vi "WBRT Main.vi"() -> ()   [LabVIEW 2012]
doc: "Whirlybird Controller\n\nAuthor: Brandon Steele\n\nCopyright: Brigham Young University"
uses:
  Custom Controls/WBRT Filter Data.ctl
  Custom Controls/WBRT Filter Type.ctl
  Custom Controls/WBRT Setpoints.ctl
  Custom Controls/WBRT Gains.ctl
  <vilib>/Platform/TimedLoop/XDataNode/timing_clust.ctl
  <vilib>/Platform/TimedLoop/XDataNode/nitl_modes.ctl
  <vilib>/Platform/TimedLoop/XDataNode/wakeup.ctl
  <vilib>/Platform/TimedLoop/XDataNode/XDataNode.xnode
  <vilib>/Platform/TimedLoop/XDataNode/XDNodeRunTimeDep.lvlib
  <vilib>/vision/NI_Vision_Development_Module.lvlib
panel:
  in  "Zero Encoders":bool
  in  "Tab Control":T1(tab)
  out "Waveform\nChart":T2(graph)={"[0]"=-46.87203500802024, "[1]"=-28.440021241425494, "[2]"=-1.368001021739454, "[3]"=0.0, "[4]"=0.0, "[5]"=0.0, "[6]"=-0.58608, "[7]"=-4.542120000000001, "[8]"=-5.347980000000001, "[9]"=-0.5018779999999999, "[10]"=0.6305, "[11]"=-0.633022}
  out "dt (msec)":u32=67
  in  "Red or Hue Range":cluster{"Lower value":i32, "Upper value":i32}={"Lower value"=150, "Upper value"=255}
  in  "Green Range":cluster{"Lower value":i32, "Upper value":i32}={"Lower value"=0, "Upper value"=255}
  in  "Blue Range":cluster{"Lower value":i32, "Upper value":i32}={"Lower value"=0, "Upper value"=255}
  in  "Pixel Format":T3(ring)=enum."160 x 120 MJPG"
  in  "Compression":u32(slide)=85 scale=0.0..99.0
  in  "Frame Rate":u32(slide)=15 max=30 scale=0.0..30.0
  in  "Camera IP address":string="192.168.0.90"
  out "Centroid":cluster{"X Centroid":sgl, "Y Centroid":sgl}={"X Centroid"=78.86318, "Y Centroid"=61.304207} {"Y Centroid" format="%.2f"; "X Centroid" format="%.2f"}
  in  "Find Centroid":bool
  out "Image":T4(plugin-control)
  out "Error Chart":T5(graph)
  in  "Auto Zero?":bool
  in  "Delay (s)":dbl=30.0
  in  "Auto Shutdown":bool
  in  "Left Motor (0-100%)":dbl
  in  "Right Motor (0-100%)":dbl
  in  "Manual Motor Control":bool
  out "Left Motor Display":dbl=-1.2876027999998882
  out "Right Motor Display":dbl=-0.09379669999989915
  in  "Lock together":bool=TRUE
  in  "Save Data":bool
  out "Array Size":i32
  in  "Filter Data":T6={"Filter Enabled?"=FALSE, "Filter Type"=enum."Equi-Ripple", "Pass Frequency"=0.45000000000000007, "Stop Frequency (Equi-Ripple)"=0.125, "Order"=2, "Ripple (dB)"=2.0} {"Stop Frequency (Equi-Ripple)" format="%0.3f"; "Pass Frequency" format="%0.3f"}
  in  "Landing Factor\n(power reduction per loop)":dbl=0.1
  in  "Enable Camera":bool
  out "Camera \nerror codes":errorcluster
  in  "Spin up time (s)":dbl=2.0
  in  "Gains":T8
  in  "Commanded Values":T9
  in  "Start":bool
  in  "Stop":bool
  out "Running":bool
  out "Late?":bool
  out "Freq (Hz)":dbl=100.0
  out "dt (msec)":u32=10
  in  "Loop Rate (Hz)":dbl=100.0
  # "Color Segmentation Thresholds"
  # "Must be set before runtime"
  # "Run Mathscript Node"
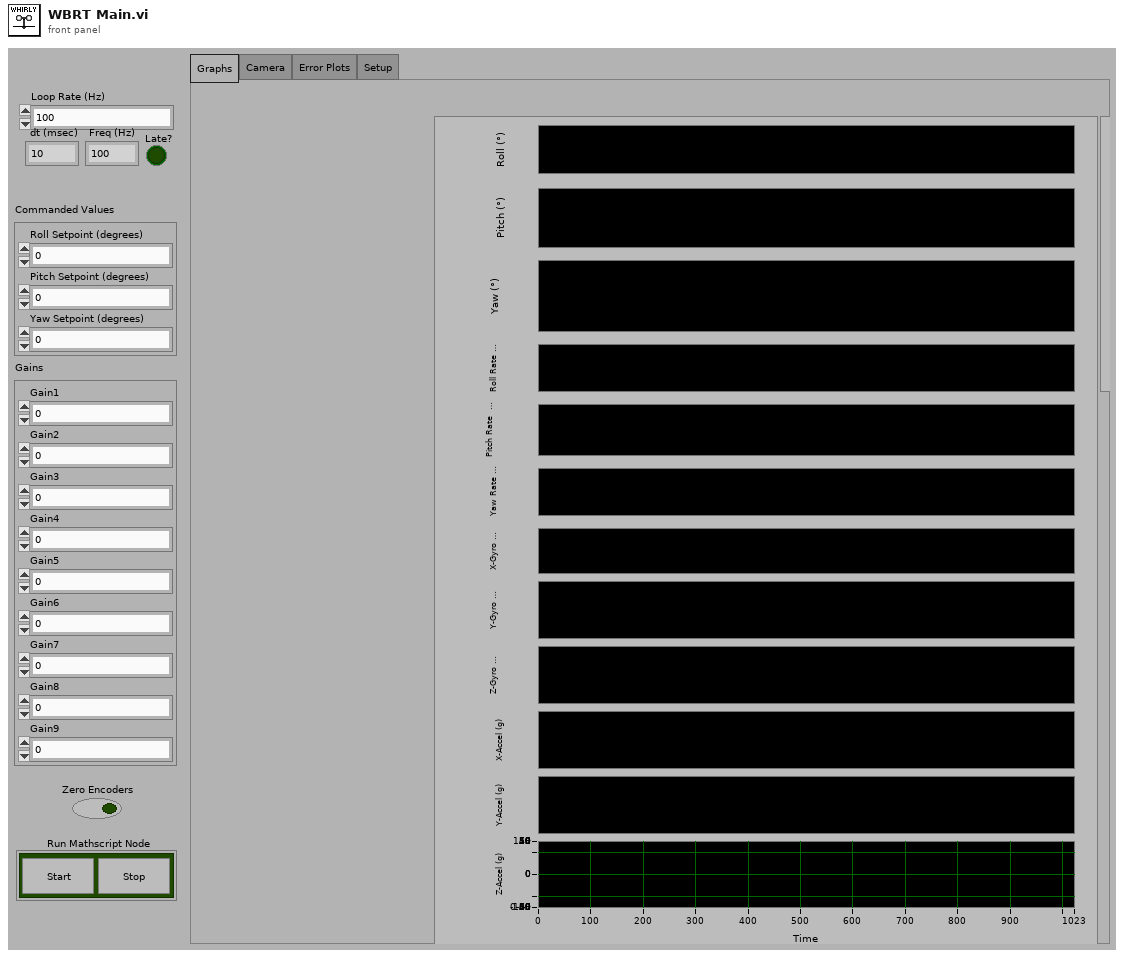
[diagram p1: front panel]
types:
  T1 = enum32{"Graphs", "Camera", "Error Plots", "Setup"}
  T2 = cluster{"[0]":dbl, "[1]":dbl, "[2]":dbl, "[3]":dbl, "[4]":dbl, "[5]":dbl, "[6]":dbl, "[7]":dbl, "[8]":dbl, "[9]":dbl, "[10]":dbl, "[11]":dbl}
  T3 = enum16{"640 x 480 MJPG", "320 x 240 MJPG", "160 x 120 MJPG"}
  T4 = typedef "IMAQ Image.ctl" = refnum<image>
  T5 = cluster{"[0]":dbl, "[1]":dbl, "[2]":dbl, "[3]":dbl}
  T6 = typedef "WBRT Filter Data.ctl" = cluster{"Filter Enabled?":bool, "Filter Type":T7, "Pass Frequency":dbl, "Stop Frequency (Equi-Ripple)":dbl, "Order":i32, "Ripple (dB)":dbl}
  T7 = typedef "WBRT Filter Type.ctl" = enum16{"Equi-Ripple", "Butterworth", "Chebyshev"}
  T8 = typedef "WBRT Gains.ctl" = cluster{"Gain1":dbl, "Gain2":dbl, "Gain3":dbl, "Gain4":dbl, "Gain5":dbl, "Gain6":dbl, "Gain7":dbl, "Gain8":dbl, "Gain9":dbl}
  T9 = typedef "WBRT Setpoints.ctl" = cluster{"Roll Setpoint (degrees)":dbl, "Pitch Setpoint (degrees)":dbl, "Yaw Setpoint (degrees)":dbl}
  T10 = typedef "XDNodeRunTimeDep.lvlib/timing_clust.ctl" = cluster{"Expected End [f-1]":u64, "Actual End [f-1]":u64, "Finished Late? [f-1]":bool, "Expected End [i-1]":u64, "Actual End [i-1]":u64, "Finished Late? [i-1]":bool, "Expected Start [i]":u64, "Actual Start [i]":u64, "Expected Start [f]":u64, "Actual Start [f]":u64, "Source Name":string, "Structure Name":string, "Period":i64, "Deadline":i64, "Offset":i64, "Start":i64, "Priority":i32, "Timeout":i32, "Mode":T11, "Wakeup Reason":T12, "Error":errorcluster, "Source Type":string, "Secondary Source Type":string, "Global End Time":u64, "Global Start Time":u64, "Frame Duration":u64, "Iteration Duration":u64, "Assigned CPU":i32, "I/O Scan Engine Mode":u32}
  T11 = typedef "XDNodeRunTimeDep.lvlib/nitl_modes.ctl" = enum32{"No Change", "Process missed periods, maintain original phase", "Discard missed periods, maintain original phase", "Process missed periods, ignore original phase", "Discard missed periods, ignore original phase"}
  T12 = typedef "XDNodeRunTimeDep.lvlib/wakeup.ctl" = enum32{"Normal", "Aborted", "Asynchronous wakeup", "Timing source error", "Timed loop error", "Timeout"}
  T13 = typedef "Image Type" = u32
  T14 = typedef "WBRT State.ctl" = cluster{"Encoders":T15, "SPI Data":T16, "Camera":cluster{"Numeric":dbl}, "Filter Data":T6, "FPGA VI Reference":T17, "dt":dbl, "Elapsed Time (msec)":u32, "Setpoints":T9, "Commands":T18, "Trajectory Data":dbl[][], "Gains":T8, "Global Variables":T19, "Centroid":cluster{"X Centroid":sgl, "Y Centroid":sgl}, "Error1":dbl, "Error2":dbl, "Error3":dbl, "Error4":dbl, "Recorded Data":dbl[][], "Landing Factor":dbl}
  T15 = typedef "WBRT Encoders.ctl" = cluster{"Roll":dbl, "Pitch":dbl, "Yaw":dbl, "Roll Trim":dbl, "Pitch Trim":dbl, "Yaw Trim":dbl, "Roll Rate":dbl, "Pitch Rate":dbl, "Yaw Rate":dbl}
  T16 = typedef "WBRT SPI Data.ctl" = cluster{"X-Gyro":dbl, "Y-Gyro":dbl, "Z-Gyro":dbl, "X-Accel":dbl, "Y-Accel":dbl, "Z-Accel":dbl}
  T17 = typedef "FPGA SPI_FPGA Ref.ctl" = refnum<k20>
  T18 = typedef "WBRT Commands.ctl" = cluster{"Left Command":dbl, "Right Command":dbl}
  T19 = typedef "WBRT Global Variables.ctl" = cluster{"Variable1":dbl[][], "Variable2":dbl[][], "Variable3":dbl[][], "Variable4":dbl[][]}
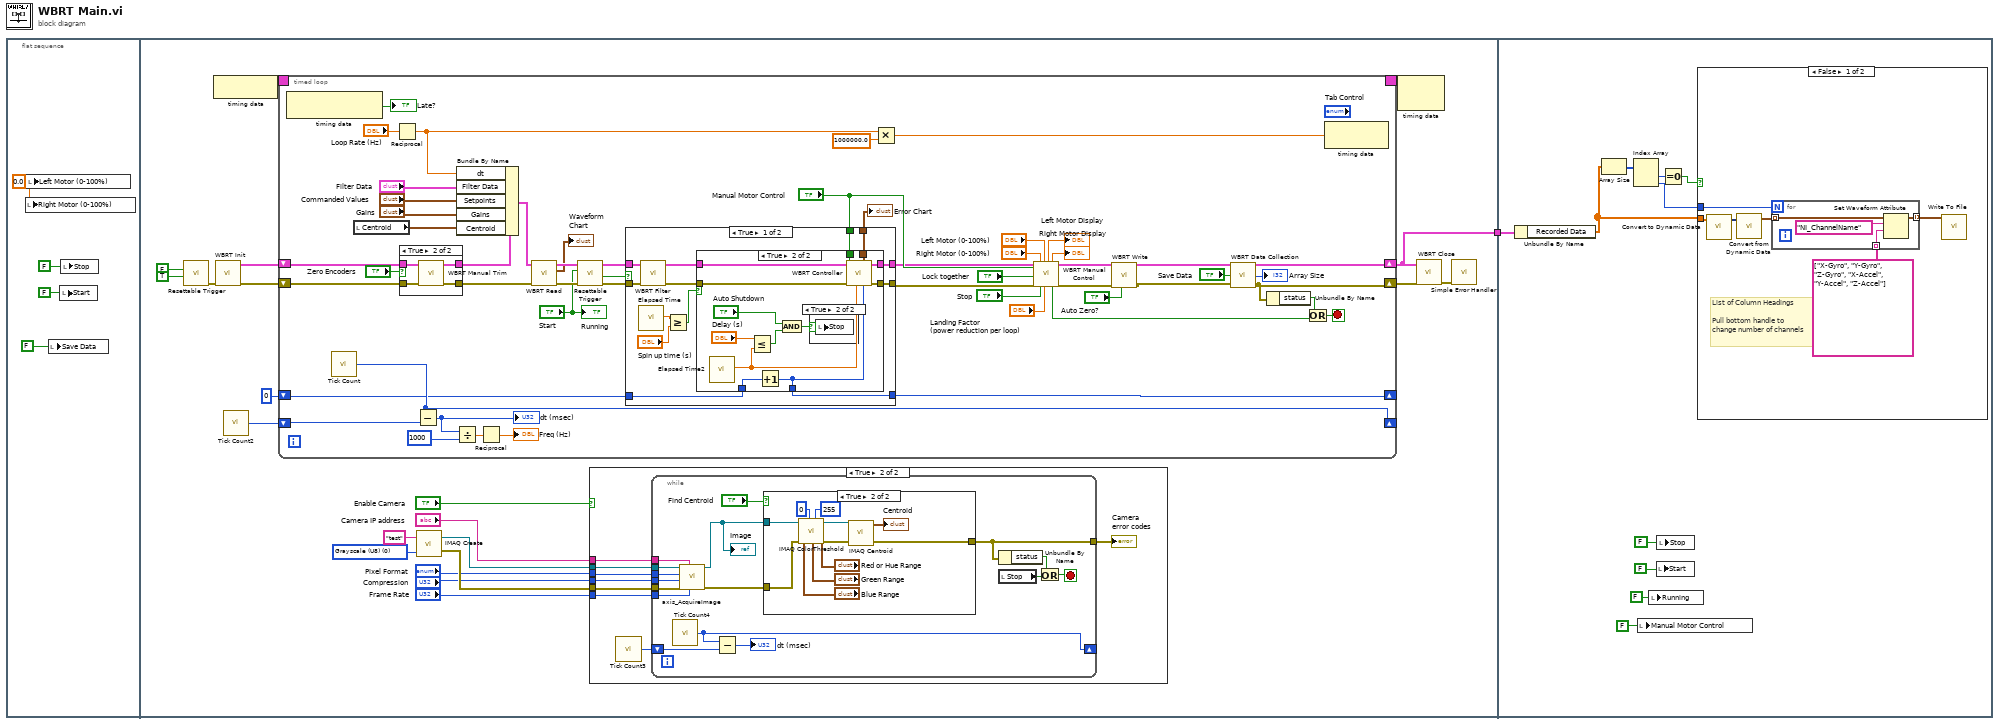
[diagram p0: block diagram]
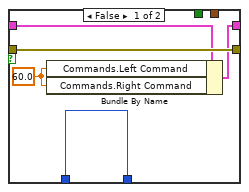
[diagram p5: hidden frame]
diagram:
  n1 = flat-sequence {
    tunnel: [w16] -> w1
    tunnel: w1 -> [w164]
    frame #0 {
      w2 = 0.0 ("Left Motor (0-100%)")
      n2 = local write "Right Motor (0-100%)"(w2) -> ()
      n3 = local write "Left Motor (0-100%)"(w2) -> ()
      n4 = local write "Save Data"(FALSE ("Camera\nOnly")) -> ()
      n5 = local write "Start"(FALSE ("Stop")) -> ()
      n6 = local write "Stop"(FALSE ("Stop")) -> ()
    }
    frame #1 {
      w14 = T13 0 items=["Grayscale (U8)", "Grayscale (I16)", "Grayscale (SGL)", "Complex (CSG)", "RGB (U32)", "HSL (U32)", "RGB (U64)", "Grayscale (U16)"] ("Image Type \n(doesn't seem to work)")
      n7 = call "Resettable Trigger.vi"("Reset (F)"=TRUE, "State"=FALSE) -> ("error out"=w19:errorcluster)  [unwired: 7 in, 2 out]
      n8 = node-c288() -> (w26:T10)
      n9 = call "WBRT Init.vi"("error in"=w19) -> ("error out"=w23:errorcluster, "WBRT State Out"=w24:T14)  [unwired: 9 in]
      n10 = call "Tick Count2"() -> ("Tick Count(mSec)"=w20:u32)
      n11 = timed-loop {
        timing: w26 -> [_]
        timing-out: [_] -> w25
        shift-right: [w88] -> w16
        shift-left: w24 -> [w70]
        shift-right: [w73] -> w22
        shift-left: w23 -> [w72]
        shift-right: [w99] -> _
        shift-left: w20 -> [w108]
        shift-right: [w65] -> _
        shift-left: 0 -> [w66]
        stop <- w110 stop-if-true
        n12 = node-c288() -> (→"Late?":bool)  [unwired: 1 in]
        n13 = call "Tick Count"() -> ("Tick Count(mSec)"=w99:u32)
        n14 = local read "Centroid"() -> (w90:cluster{"X Centroid":sgl, "Y Centroid":sgl})
        n15 = Reciprocal(x="Loop Rate (Hz)") -> (1/x=w95:dbl)
        n16 = case shown="True" "Zero Encoders" {
          tunnel: w72 -> [w116 w120]
          tunnel: [w116 w119] -> w71
          tunnel: w70 -> [w115 w118]
          tunnel: [w115 w117] -> w69
          frame False {
          }
          frame True {
            n17 = call "WBRT Manual Trim.vi"("error in"=w120, "WBRT State in"=w118) -> ("error out"=w119:errorcluster, "WBRT State Out"=w117:T14)  [unwired: 8 in]
          }
        }
        n18 = Subtract(x=w99, y=w108) -> (x-y=w107:u32)
        "dt (msec)" <- w107
        n19 = Divide(x=w107, y=u32 1000) -> (x/y=w105:dbl)
        n20 = Bundle By Name(cluster=w69, "dt"=w95, "Filter Data"="Filter Data", "Setpoints"="Commanded Values", "Gains"="Gains", "Centroid"=w90) -> (w103:T14)
        n21 = Reciprocal(x=w105) -> (1/x=→"Freq (Hz)":dbl)
        n22 = call "WBRT Read.vi"("error in"=w71, "WBRT State In"=w103) -> ("error out"=w98:errorcluster, "Chart Data"=→"Waveform\nChart":T2, "WBRT State Out"=w114:T14)  [unwired: 7 in]
        n23 = call "Resettable Trigger.vi"("error in (no error)"=w98, "State"="Start") -> ("error out"=w97:errorcluster, "Triggered?"=w96:bool)  [unwired: 7 in, 1 out]
        n24 = case shown="True" w96 {
          tunnel: w114 -> [w133 w155]
          tunnel: [w128 w154] -> w76
          tunnel: [w129 w155] -> w77
          tunnel: w97 -> [w130 w154]
          tunnel: "Manual Motor Control" -> [w127 _]
          tunnel: w66 -> [w123 w153]
          tunnel: [w122 w153] -> w65
          tunnel: [w121 _] -> w64
          frame True {
            n25 = call "Elapsed Time"() -> ("Elapsed Time (s)"=w126:dbl)  [unwired: 12 in, 7 out]
            n26 = call "WBRT Filter.vi"("error in (no error)"=w130, "WBRT State In"=w133) -> ("error out"=w131:errorcluster, "WBRT State Out"=w132:T14)  [unwired: 8 in]
            n27 = Greater Or Equal?(x=w126, y="Spin up time (s)") -> (x >= y?=w124:bool)
            n28 = case shown="True" w124 {
              tunnel: w132 -> [w137 w151]
              tunnel: w131 -> [w138 w150]
              tunnel: [w136 w149] -> w129
              tunnel: [w138 w148] -> w128
              tunnel: w127 -> [_ w147]
              tunnel: w123 -> [w134 w146]
              tunnel: [w134 w145] -> w122
              tunnel: [_ w139] -> w121
              frame False {
                w135 = 60.0 ("Commands.Left Command")
                n29 = Bundle By Name(cluster=w137, "Commands.Left Command"=w135, "Commands.Right Command"=w135) -> (w136:T14)
              }
              frame True {
                n30 = call "Elapsed Time2"() -> ("Elapsed Time (s)"=w141:dbl)  [unwired: 12 in, 7 out]
                n31 = Less Or Equal?(x="Delay (s)", y=w141) -> (x <= y?=w144:bool)
                n32 = Increment(x=w146) -> (x+1=w145:i32)
                n33 = And(x="Auto Shutdown", y=w144) -> (x .and. y?=w140:bool)
                n34 = case shown="True" w140 {
                  selector: w140 -> [_ w152]
                  frame False {
                  }
                  frame True {
                    n35 = local write "Stop"(w152) -> ()
                  }
                }
                n36 = call "WBRT Controller.vi"("Loop count"=w145, "Elapsed Time"=w141, "Manual Motor Control"=w147, "error in (no error)"=w150, "WBRT State In"=w151) -> ("error out"=w148:errorcluster, "WBRT State Out"=w149:T14, "Error Chart Cluster"=w139:T5)  [unwired: 4 in]
              }
            }
          }
          frame False {
          }
        }
        "Error Chart" <- w64
        n37 = Multiply(x=w95, y=1000000.0) -> (x*y=w112:dbl)
        n38 = call "WBRT Manual Control.vi"("WBRT State In"=w77, "Manual Motor Control"="Manual Motor Control", "Lock together"="Lock together", "error in (no error)"=w76, "Right Motor (0-100%)"="Right Motor (0-100%)", "Stop In"="Stop", "Left Motor (0-100%)"="Left Motor (0-100%)", "Landing Factor"="Landing Factor\n(power reduction per loop)") -> ("Left Motor Display"=→"Left Motor Display":dbl, "Right Motor Display"=→"Right Motor Display":dbl, "Stop Out"=w85:bool, "WBRT State Out"=w87:T14, "error out"=w75:errorcluster)  [unwired: 7 in]
        n39 = call "WBRT Write.vi"("Auto Zero?"="Auto Zero?", "error in (no error)"=w75, "WBRT State In"=w87) -> ("error out"=w74:errorcluster, "WBRT State Out"=w67:T14)  [unwired: 7 in]
        n40 = call "WBRT Data Collection.vi"("error in (no error)"=w74, "Save Data"="Save Data", "WBRT State In"=w67) -> ("error out"=w73:errorcluster, "Array Size"=→"Array Size":i32, "WBRT State Out"=w88:T14)
        n41 = Unbundle By Name(w73) -> ("status"=w109:bool)
        n42 = Or(x=w109, y=w85) -> (x .or. y?=w110:bool)
        n43 = node-c288(w112) -> ()  [unwired: 1 out]
        "Running" <- "Start"
      }
      n44 = call "IMAQ Create"("Image Name"="test", "Image Type"=w14) -> ("New Image"=w11:T4, "error out"=w9:errorcluster)  [unwired: 2 in, 1 out]
      n45 = case shown="True" "Enable Camera" {
        tunnel: "Camera IP address" -> [_ w33]
        tunnel: w11 -> [_ w32]
        tunnel: "Frame Rate" -> [_ w31]
        tunnel: w9 -> [_ w30]
        tunnel: "Compression" -> [_ w29]
        tunnel: "Pixel Format" -> [_ w28]
        frame False {
        }
        frame True {
          n46 = call "Tick Count3"() -> ("Tick Count(mSec)"=w27:u32)
          n47 = while {
            tunnel: w33 -> [w49]
            tunnel: w32 -> [w50]
            tunnel: [w36] -> w34
            tunnel: w30 -> [w44]
            tunnel: w31 -> [w48]
            tunnel: w29 -> [w43]
            tunnel: w28 -> [w42]
            shift-right: [w41] -> _
            shift-left: w27 -> [w40]
            stop <- w46 stop-if-true
            n48 = call "Tick Count4"() -> ("Tick Count(mSec)"=w41:u32)
            n49 = call "axis_AcquireImage.vi"("Frame Rate"=w48, "address"=w49, "error in (no error)"=w44, "Compression"=w43, "Pixel Format"=w42, "Image In"=w50) -> ("error out"=w37:errorcluster, "Image Out"=w35:T4)  [unwired: 1 in, 3 out]
            "Image" <- w35
            n50 = Subtract(x=w41, y=w40) -> (x-y=→"dt (msec)":u32)
            n51 = case shown="True" "Find Centroid" {
              tunnel: w35 -> [_ w52]
              tunnel: w37 -> [w51 w55]
              tunnel: [w51 w53] -> w36
              frame False {
              }
              frame True {
                n52 = call "IMAQ ColorThreshold"("Blue or Luma or Val or Inten Range"="Blue Range", "Replace Value"=255 ("Replace value"), "Green or Sat Range"="Green Range", "Color Mode"=0, "error in (no error)"=w55, "Red or Hue Range"="Red or Hue Range", "Image Src"=w52) -> ("error out"=w54:errorcluster, "Image Dst Out"=w57:T4)  [unwired: 3 in]
                n53 = call "IMAQ Centroid"("error in (no error)"=w54, "Image"=w57) -> ("error out"=w53:errorcluster, "Centroid"=→"Centroid":cluster{"X Centroid":sgl, "Y Centroid":sgl})  [unwired: 2 in]
              }
            }
            n54 = Unbundle By Name(w36) -> ("status"=w47:bool)
            n55 = local read "Stop"() -> (w45:bool)
            n56 = Or(x=w47, y=w45) -> (x .or. y?=w46:bool)
          }
          "Camera \nerror codes" <- w34
        }
      }
      n57 = node-c288(w25) -> ()  [unwired: 1 out]
      n58 = call "WBRT Close.vi"("error in"=w22, "WBRT State In"=w16) -> ("error out"=w21:errorcluster)  [unwired: 9 in]
      n59 = call <vilib>:"Simple Error Handler.vi"("error in (no error)"=w21) -> ()  [unwired: 4 in, 5 out]
    }
    frame #2 {
      n60 = Unbundle By Name(w164) -> ("Recorded Data"=w163:dbl[][])
      n61 = Array Size(array=w163) -> (size(s)=w168:i32[])
      n62 = Index Array(array=w168) -> (element #1=w167:i32, element #2=w165:i32)  [unwired: 2 in]
      n63 = local write "Manual Motor Control"(FALSE ("Stop")) -> ()
      n64 = local write "Running"(FALSE ("Stop")) -> ()
      n65 = local write "Start"(FALSE ("Stop")) -> ()
      n66 = local write "Stop"(FALSE ("Stop")) -> ()
      n67 = Equal To 0?(x=w167) -> (x = 0?=w166:bool)
      n68 = case shown="False" w166 {
        tunnel: w163 -> [w178 _]
        tunnel: w165 -> [w173 _]
        frame False {
          # "List of Column Headings\n\nPull bottom handle to\nchange number of channels"
          n69 = call "Convert to Dynamic Data"("2D Array"=w178) -> ("Dynamic Data Type"=w177:dynamicdata)  [unwired: 3 in]
          n70 = call "Convert from Dynamic Data"("Dynamic Data Type"=w177) -> ("Array of Waveform"=w176:waveform(dbl)[])  [unwired: 3 in]
          n71 = for {
            N: w173 -> [_]
            tunnel: w176 -> [w182] mode=indexing
            tunnel: string[] ["X-Gyro", "Y-Gyro", "Z-Gyro", "X-Accel", "Y-Accel", "Z-Accel"] ("Array") -> [w179] mode=indexing
            tunnel: [w181] -> w174 mode=indexing
            n72 = Set Waveform Attribute(5:w179, 6:"NI_ChannelName" ("name"), 7:w182) -> (3:w181:waveform(dbl))  [unwired: 1 in, 2 out]
          }
          n73 = call "Write To File"("Signals"=w174) -> ()  [unwired: 16 in, 3 out]
        }
        frame True {
        }
      }
    }
  }
